vi "UNSUBSCRIBE.vi"(0 "TCP session out":refnum<k5>, 5 "Channels":string[](array[string]), 11 "error in":errorcluster) -> (4 "TCP session out":refnum<k5>, 6 "Data":T1, 15 "error out":errorcluster)   [LabVIEW 2023]
uses:
  SubVIs/Controls/redis-data.ctl
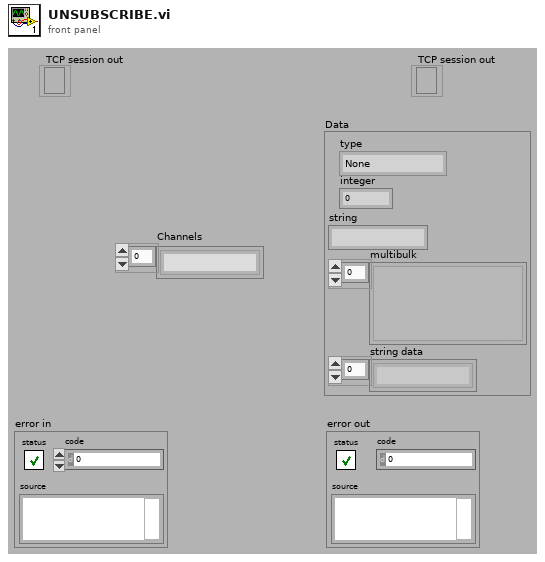
[diagram p1: front panel]
types:
  T1 = typedef "redis-data.ctl" = cluster{"type":enum16{"None", "Error", "Status", "Nil", "Integer", "String", "Multibulk"}, "integer":i64, "string":string, "multibulk":variant[], "string data":string[]}
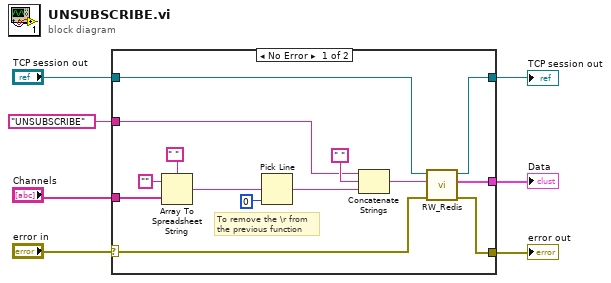
[diagram p0: block diagram]
diagram:
  n1 = case shown="No Error" "error in" {
    selector: "error in" -> [w12 w23]
    tunnel: "Channels" -> [w21 _]
    tunnel: "UNSUBSCRIBE" -> [w14 _]
    tunnel: "TCP session out" -> [w9 w22]
    tunnel: [w11 w23] -> w3
    tunnel: [w10 _] -> w2
    tunnel: [w8 w22] -> w1
    frame No Error {
      # "To remove the \\r from\nthe previous function"
      n2 = Array To Spreadsheet String(delimiter (Tab)=" ", array=w21, 3:"" ("format string")) -> (spreadsheet string=w16:string)
      n3 = Pick Line(multi-line string=w16, line index=0) -> (output string=w17:string)  [unwired: 1 in]
      n4 = Concatenate Strings(w14, " ", w17) -> (w13:string)
      n5 = call "RW_Redis.vi"("error in"=w12, "command"=w13, "TCP session in"=w9) -> ("error out"=w11:errorcluster, "Data"=w10:T1, "TCP session out"=w8:refnum<k5>)  [unwired: 6 in]
    }
    frame Error {
    }
  }
  "error out" <- w3
  "Data" <- w2
  "TCP session out" <- w1
